vi "LHPulse.vi"(2 "LHPulse(us)":T1, 3 "LHHeizen?":T2) -> ()   [LabVIEW 2010]
uses:
  <vilib>/eio/EIONode/EIONode.xnode
  <vilib>/rvi/eio/nirviEIOImplementation/nirviEIOImplementation.xnode
  <vilib>/rvi/eio/common/nirviEmuClasses.ctl
  <vilib>/rvi/eio/common/nirviEmuTemplateMethod_noerrors.vi
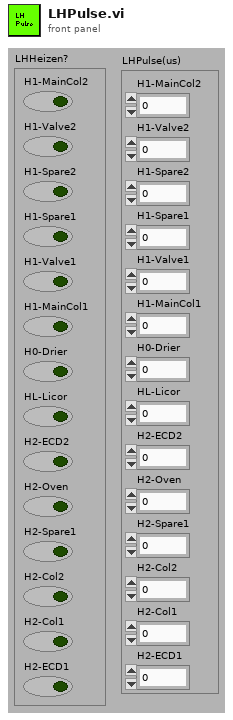
[diagram p1: front panel]
types:
  T1 = cluster{"H1-MainCol2":u32, "H1-Valve2":u32, "H1-Spare2":u32, "H1-Spare1":u32, "H1-Valve1":u32, "H1-MainCol1":u32, "H0-Drier":u32, "HL-Licor":u32, "H2-ECD2":u32, "H2-Oven":u32, "H2-Spare1":u32, "H2-Col2":u32, "H2-Col1":u32, "H2-ECD1":u32}
  T2 = cluster{"H1-MainCol2":bool, "H1-Valve2":bool, "H1-Spare2":bool, "H1-Spare1":bool, "H1-Valve1":bool, "H1-MainCol1":bool, "H0-Drier":bool, "HL-Licor":bool, "H2-ECD2":bool, "H2-Oven":bool, "H2-Spare1":bool, "H2-Col2":bool, "H2-Col1":bool, "H2-ECD1":bool}
  T3 = typedef "nirviEmuClasses.ctl" = enum16{"IO Read", "IO Write", "Method", "Property Read", "Property Write"}
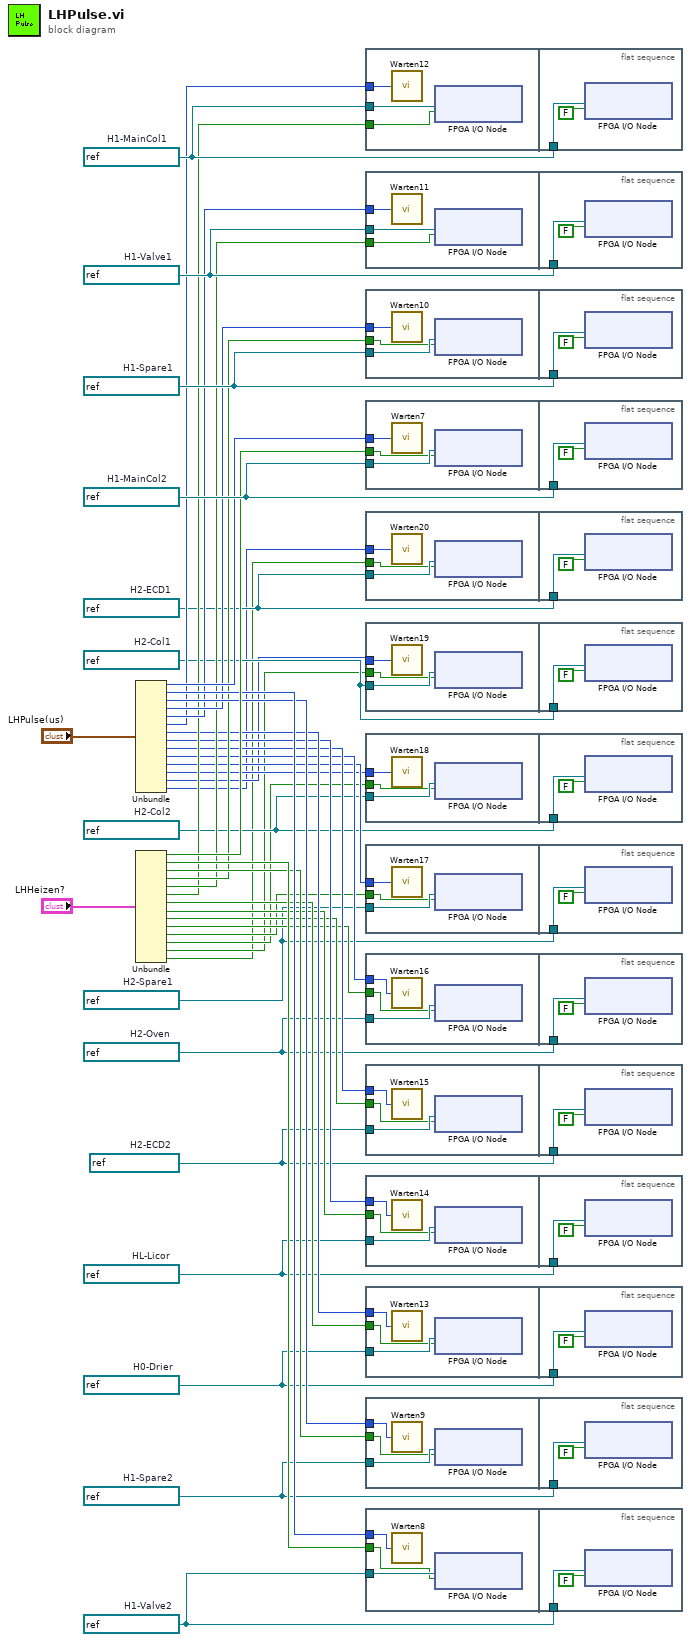
[diagram p0: block diagram]
diagram:
  w5 = refnum<k21> "Mod5/DIO20"  # H2-ECD1
  w8 = refnum<k21> "Mod5/DIO19"  # H2-Col1
  w11 = refnum<k21> "Mod5/DIO18"  # H2-Col2
  w14 = refnum<k21> "Mod5/DIO17"  # H2-Spare1
  w17 = refnum<k21> "Mod5/DIO16"  # H2-Oven
  w20 = refnum<k21> "Mod5/DIO1"  # H2-ECD2
  w23 = refnum<k21> "Mod5/DIO27"  # HL-Licor
  w26 = refnum<k21> "Mod5/DIO11"  # H0-Drier
  w29 = refnum<k21> "Mod6/DIO28"  # H1-MainCol1
  w32 = refnum<k21> "Mod6/DIO27"  # H1-Valve1
  w35 = refnum<k21> "Mod6/DIO26"  # H1-Spare1
  w38 = refnum<k21> "Mod6/DIO25"  # H1-Spare2
  w39 = refnum<k21> "Mod6/DIO24"  # H1-Valve2
  w44 = refnum<k21> "Mod6/DIO17"  # H1-MainCol2
  n1 = Unbundle("LHPulse(us)") -> ("H1-MainCol2"=w42:u32, "H1-Valve2"=w40:u32, "H1-Spare2"=w36:u32, "H1-Spare1"=w33:u32, "H1-Valve1"=w31:u32, "H1-MainCol1"=w27:u32, "H0-Drier"=w24:u32, "HL-Licor"=w21:u32, "H2-ECD2"=w18:u32, "H2-Oven"=w15:u32, "H2-Spare1"=w12:u32, "H2-Col2"=w9:u32, "H2-Col1"=w6:u32, "H2-ECD1"=w3:u32)
  n2 = Unbundle("LHHeizen?") -> ("H1-MainCol2"=w43:bool, "H1-Valve2"=w41:bool, "H1-Spare2"=w37:bool, "H1-Spare1"=w34:bool, "H1-Valve1"=w30:bool, "H1-MainCol1"=w28:bool, "H0-Drier"=w25:bool, "HL-Licor"=w22:bool, "H2-ECD2"=w19:bool, "H2-Oven"=w16:bool, "H2-Spare1"=w13:bool, "H2-Col2"=w10:bool, "H2-Col1"=w7:bool, "H2-ECD1"=w4:bool)
  n3 = flat-sequence {
    tunnel: w29 -> [w47]
    tunnel: w28 -> [w46]
    tunnel: w27 -> [w45]
    tunnel: w29 -> [w60]
    frame #0 {
      n4 = call "Warten12"("Count(uSec)"=w45) -> ()  [unwired: 1 out]
      n5 = xnode "FPGA I/O Node"("I/O Item"=w46, "FPGA I/O In"=w47) -> ()  [unwired: 1 out]
    }
    frame #1 {
      n6 = xnode "FPGA I/O Node"("I/O Item"=FALSE, "FPGA I/O In"=w60) -> ()  [unwired: 1 out]
    }
  }
  n7 = flat-sequence {
    tunnel: w32 -> [w74]
    tunnel: w30 -> [w73]
    tunnel: w31 -> [w72]
    tunnel: w32 -> [w87]
    frame #0 {
      n8 = call "Warten11"("Count(uSec)"=w72) -> ()  [unwired: 1 out]
      n9 = xnode "FPGA I/O Node"("I/O Item"=w73, "FPGA I/O In"=w74) -> ()  [unwired: 1 out]
    }
    frame #1 {
      n10 = xnode "FPGA I/O Node"("I/O Item"=FALSE, "FPGA I/O In"=w87) -> ()  [unwired: 1 out]
    }
  }
  n11 = flat-sequence {
    tunnel: w35 -> [w101]
    tunnel: w34 -> [w100]
    tunnel: w33 -> [w99]
    tunnel: w35 -> [w114]
    frame #0 {
      n12 = call "Warten10"("Count(uSec)"=w99) -> ()  [unwired: 1 out]
      n13 = xnode "FPGA I/O Node"("I/O Item"=w100, "FPGA I/O In"=w101) -> ()  [unwired: 1 out]
    }
    frame #1 {
      n14 = xnode "FPGA I/O Node"("I/O Item"=FALSE, "FPGA I/O In"=w114) -> ()  [unwired: 1 out]
    }
  }
  n15 = flat-sequence {
    tunnel: w44 -> [w128]
    tunnel: w43 -> [w127]
    tunnel: w42 -> [w126]
    tunnel: w44 -> [w141]
    frame #0 {
      n16 = call "Warten7"("Count(uSec)"=w126) -> ()  [unwired: 1 out]
      n17 = xnode "FPGA I/O Node"("I/O Item"=w127, "FPGA I/O In"=w128) -> ()  [unwired: 1 out]
    }
    frame #1 {
      n18 = xnode "FPGA I/O Node"("I/O Item"=FALSE, "FPGA I/O In"=w141) -> ()  [unwired: 1 out]
    }
  }
  n19 = flat-sequence {
    tunnel: w5 -> [w155]
    tunnel: w4 -> [w154]
    tunnel: w3 -> [w153]
    tunnel: w5 -> [w168]
    frame #0 {
      n20 = call "Warten20"("Count(uSec)"=w153) -> ()  [unwired: 1 out]
      n21 = xnode "FPGA I/O Node"("I/O Item"=w154, "FPGA I/O In"=w155) -> ()  [unwired: 1 out]
    }
    frame #1 {
      n22 = xnode "FPGA I/O Node"("I/O Item"=FALSE, "FPGA I/O In"=w168) -> ()  [unwired: 1 out]
    }
  }
  n23 = flat-sequence {
    tunnel: w8 -> [w182]
    tunnel: w7 -> [w181]
    tunnel: w6 -> [w180]
    tunnel: w8 -> [w195]
    frame #0 {
      n24 = call "Warten19"("Count(uSec)"=w180) -> ()  [unwired: 1 out]
      n25 = xnode "FPGA I/O Node"("I/O Item"=w181, "FPGA I/O In"=w182) -> ()  [unwired: 1 out]
    }
    frame #1 {
      n26 = xnode "FPGA I/O Node"("I/O Item"=FALSE, "FPGA I/O In"=w195) -> ()  [unwired: 1 out]
    }
  }
  n27 = flat-sequence {
    tunnel: w11 -> [w209]
    tunnel: w10 -> [w208]
    tunnel: w9 -> [w207]
    tunnel: w11 -> [w222]
    frame #0 {
      n28 = call "Warten18"("Count(uSec)"=w207) -> ()  [unwired: 1 out]
      n29 = xnode "FPGA I/O Node"("I/O Item"=w208, "FPGA I/O In"=w209) -> ()  [unwired: 1 out]
    }
    frame #1 {
      n30 = xnode "FPGA I/O Node"("I/O Item"=FALSE, "FPGA I/O In"=w222) -> ()  [unwired: 1 out]
    }
  }
  n31 = flat-sequence {
    tunnel: w14 -> [w236]
    tunnel: w13 -> [w235]
    tunnel: w12 -> [w234]
    tunnel: w14 -> [w249]
    frame #0 {
      n32 = call "Warten17"("Count(uSec)"=w234) -> ()  [unwired: 1 out]
      n33 = xnode "FPGA I/O Node"("I/O Item"=w235, "FPGA I/O In"=w236) -> ()  [unwired: 1 out]
    }
    frame #1 {
      n34 = xnode "FPGA I/O Node"("I/O Item"=FALSE, "FPGA I/O In"=w249) -> ()  [unwired: 1 out]
    }
  }
  n35 = flat-sequence {
    tunnel: w17 -> [w263]
    tunnel: w16 -> [w262]
    tunnel: w15 -> [w261]
    tunnel: w17 -> [w276]
    frame #0 {
      n36 = call "Warten16"("Count(uSec)"=w261) -> ()  [unwired: 1 out]
      n37 = xnode "FPGA I/O Node"("I/O Item"=w262, "FPGA I/O In"=w263) -> ()  [unwired: 1 out]
    }
    frame #1 {
      n38 = xnode "FPGA I/O Node"("I/O Item"=FALSE, "FPGA I/O In"=w276) -> ()  [unwired: 1 out]
    }
  }
  n39 = flat-sequence {
    tunnel: w20 -> [w290]
    tunnel: w19 -> [w289]
    tunnel: w18 -> [w288]
    tunnel: w20 -> [w303]
    frame #0 {
      n40 = call "Warten15"("Count(uSec)"=w288) -> ()  [unwired: 1 out]
      n41 = xnode "FPGA I/O Node"("I/O Item"=w289, "FPGA I/O In"=w290) -> ()  [unwired: 1 out]
    }
    frame #1 {
      n42 = xnode "FPGA I/O Node"("I/O Item"=FALSE, "FPGA I/O In"=w303) -> ()  [unwired: 1 out]
    }
  }
  n43 = flat-sequence {
    tunnel: w23 -> [w317]
    tunnel: w22 -> [w316]
    tunnel: w21 -> [w315]
    tunnel: w23 -> [w330]
    frame #0 {
      n44 = call "Warten14"("Count(uSec)"=w315) -> ()  [unwired: 1 out]
      n45 = xnode "FPGA I/O Node"("I/O Item"=w316, "FPGA I/O In"=w317) -> ()  [unwired: 1 out]
    }
    frame #1 {
      n46 = xnode "FPGA I/O Node"("I/O Item"=FALSE, "FPGA I/O In"=w330) -> ()  [unwired: 1 out]
    }
  }
  n47 = flat-sequence {
    tunnel: w26 -> [w344]
    tunnel: w25 -> [w343]
    tunnel: w24 -> [w342]
    tunnel: w26 -> [w357]
    frame #0 {
      n48 = call "Warten13"("Count(uSec)"=w342) -> ()  [unwired: 1 out]
      n49 = xnode "FPGA I/O Node"("I/O Item"=w343, "FPGA I/O In"=w344) -> ()  [unwired: 1 out]
    }
    frame #1 {
      n50 = xnode "FPGA I/O Node"("I/O Item"=FALSE, "FPGA I/O In"=w357) -> ()  [unwired: 1 out]
    }
  }
  n51 = flat-sequence {
    tunnel: w38 -> [w371]
    tunnel: w37 -> [w370]
    tunnel: w36 -> [w369]
    tunnel: w38 -> [w384]
    frame #0 {
      n52 = call "Warten9"("Count(uSec)"=w369) -> ()  [unwired: 1 out]
      n53 = xnode "FPGA I/O Node"("I/O Item"=w370, "FPGA I/O In"=w371) -> ()  [unwired: 1 out]
    }
    frame #1 {
      n54 = xnode "FPGA I/O Node"("I/O Item"=FALSE, "FPGA I/O In"=w384) -> ()  [unwired: 1 out]
    }
  }
  n55 = flat-sequence {
    tunnel: w39 -> [w398]
    tunnel: w41 -> [w397]
    tunnel: w40 -> [w396]
    tunnel: w39 -> [w411]
    frame #0 {
      n56 = call "Warten8"("Count(uSec)"=w396) -> ()  [unwired: 1 out]
      n57 = xnode "FPGA I/O Node"("I/O Item"=w397, "FPGA I/O In"=w398) -> ()  [unwired: 1 out]
    }
    frame #1 {
      n58 = xnode "FPGA I/O Node"("I/O Item"=FALSE, "FPGA I/O In"=w411) -> ()  [unwired: 1 out]
    }
  }
